vi "Coerced xy and encoders.vi"(8 "x":dbl, 9 "y":dbl) -> (0 "Red encoder":dbl, 1 "Blue encoder":dbl, 2 "Coerced X":dbl, 3 "Coerced Y":dbl)   [LabVIEW 2020]
uses:
  Robot Global Data.vi
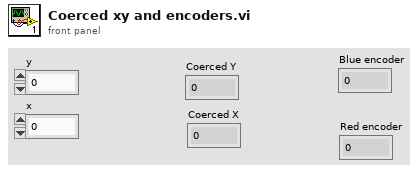
[diagram p1: front panel]
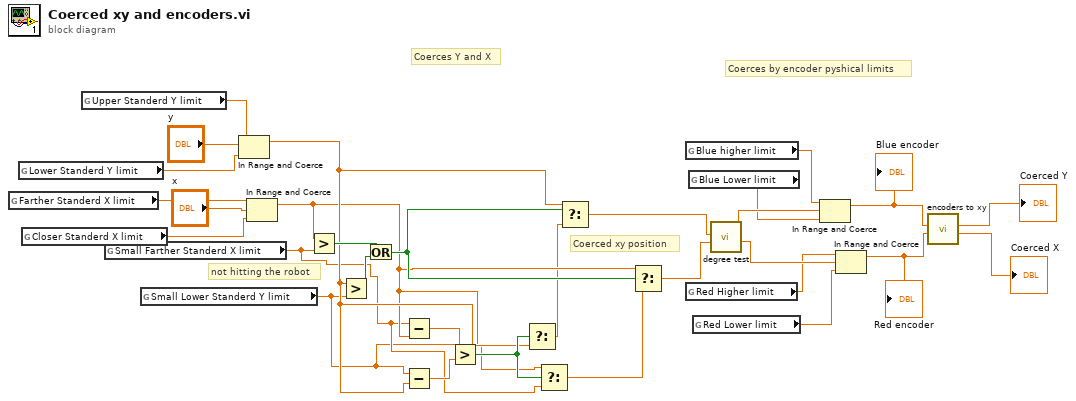
[diagram p0: block diagram]
diagram:
  # "Coerces by encoder pyshical limits"
  # "Coerces Y and X"
  # "Coerced xy position"
  # "not hitting the robot"
  n1 = global read "Robot Global Data.vi" "Farther Standerd X limit"() -> (w10:dbl)
  n2 = global read "Robot Global Data.vi" "Lower Standerd Y limit"() -> (w11:dbl)
  n3 = global read "Robot Global Data.vi" "Closer Standerd X limit"() -> (w9:dbl)
  n4 = global read "Robot Global Data.vi" "Upper Standerd Y limit"() -> (w12:dbl)
  n5 = global read "Robot Global Data.vi" "Small Farther Standerd X limit"() -> (w8:dbl)
  n6 = global read "Robot Global Data.vi" "Small Lower Standerd Y limit"() -> (w7:dbl)
  n7 = In Range and Coerce(upper limit=w12, x="y", lower limit=w11) -> (coerced(x)=w22:dbl)  [unwired: 1 out]
  n8 = In Range and Coerce(upper limit=w10, x="x", lower limit=w9) -> (coerced(x)=w21:dbl)  [unwired: 1 out]
  n9 = Greater?(x=w21, y=w8) -> (0:w27:bool)
  n10 = Greater?(x=w22, y=w7) -> (0:w28:bool)
  n11 = Or(x=w27, y=w28) -> (x .or. y?=w26:bool)
  n12 = Subtract(x=w8, y=w21) -> (x-y=w24:dbl)
  n13 = Subtract(x=w7, y=w22) -> (x-y=w25:dbl)
  n14 = Greater?(x=w24, y=w25) -> (0:w23:bool)
  n15 = Select(t=w7, s=w23, f=w22) -> (s? t:f=w19:dbl)
  n16 = Select(t=w21, s=w23, f=w8) -> (s? t:f=w20:dbl)
  n17 = Select(t=w22, s=w26, f=w19) -> (s? t:f=w15:dbl)
  n18 = Select(t=w21, s=w26, f=w20) -> (s? t:f=w18:dbl)
  n19 = global read "Robot Global Data.vi" "Blue higher limit"() -> (w5:dbl)
  n20 = global read "Robot Global Data.vi" "Red Higher limit"() -> (w4:dbl)
  n21 = global read "Robot Global Data.vi" "Blue Lower limit"() -> (w6:dbl)
  n22 = global read "Robot Global Data.vi" "Red Lower limit"() -> (w3:dbl)
  n23 = call "degree test.vi"("x"=w18, "y"=w15) -> ("red encoder"=w16:dbl, "blue encoder"=w17:dbl)  [unwired: 8 in]
  n24 = In Range and Coerce(upper limit=w5, x=w17, lower limit=w6) -> (coerced(x)=w13:dbl)  [unwired: 1 out]
  "Blue encoder" <- w13
  n25 = In Range and Coerce(upper limit=w4, x=w16, lower limit=w3) -> (coerced(x)=w14:dbl)  [unwired: 1 out]
  "Red encoder" <- w14
  n26 = call "encoders to xy.vi"("Red encoder"=w14, "Blue encoder"=w13) -> ("X"=→"Coerced X":dbl, "Y"=→"Coerced Y":dbl)  [unwired: 8 in]
